vi "Load Interpolation Table.vi"(10 "File In":path, 11 "Object Name":string) -> (0 "error out":errorcluster, 1 "Reference":dbl[](array[numeric])=[40.0, -60.0, 0.0, 65.0, 0.0, 70.0, 0.0], 2 "Table":dbl[][](array[numeric]), 3 "File":path)   [LabVIEW 2013]
uses:
  ROS/Code/SubVIs/BaxterSide.ctl
  <vilib>/Utility/config.llb/Read Key (String).vi
  <vilib>/Utility/config.llb/NI_LVConfig.lvlib
panel:
  in  "side":T1=enum."right"
  # "Object X       ObjectY         ObjectZ        ObjectA         BaseX           BaseY           BaseZ          BaseA"
  # "Far Left"
  # "Far Right"
  # "Near Left"
  # "Near Right"
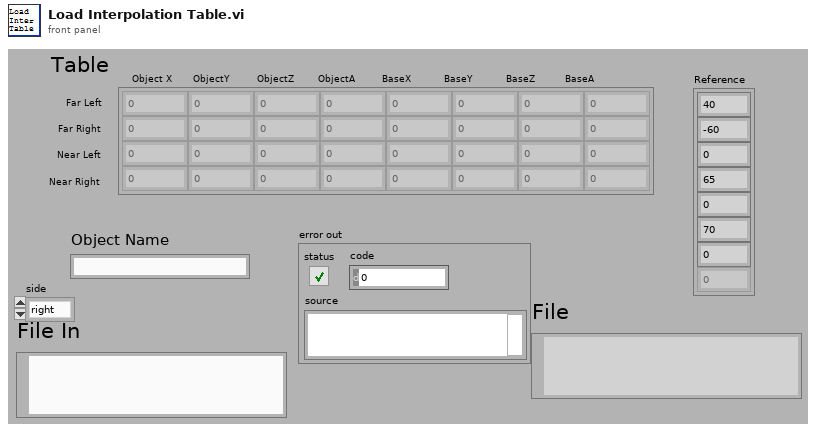
[diagram p1: front panel]
types:
  T1 = typedef "BaxterSide.ctl" = enum16{"left", "right"}
  T2 = typedef "NI_LVConfig.lvlib/Config Data RefNum.ctl" = refnum<k1>
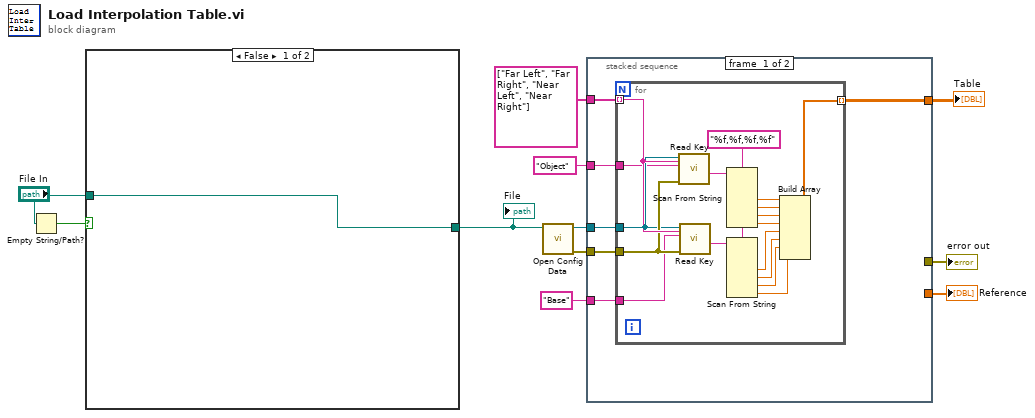
[diagram p0: block diagram]
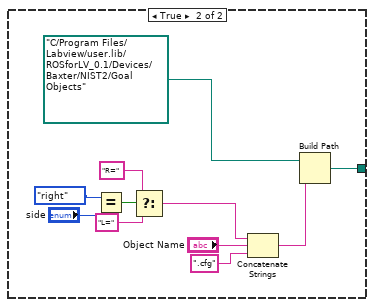
[diagram p2: hidden frame]
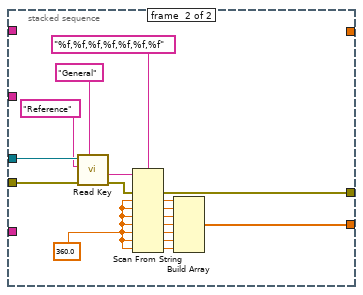
[diagram p3: hidden frame]
diagram:
  n1 = Empty String/Path?(string/path="File In") -> (empty?=w3:bool)
  n2 = case shown="False" w3 {
    tunnel: [w12 w23] -> w1
    tunnel: "File In" -> [w12 _]
    frame False {
    }
    frame True {
      n3 = Equal?(x=BaxterSide."right" ("Side"), y="side") -> (x = y?=w16:bool)
      n4 = Select(t="R=", s=w16, f="L=") -> (s? t:f=w15:string)
      n5 = Concatenate Strings(w15, "Object Name", ".cfg" ("replace string (\"\")")) -> (w20:string)
      n6 = Build Path(base path=path "C:/Program Files/Labview/user.lib/ROSforLV_0.1/Devices/Baxter/NIST2/Goal Objects", name or relative path=w20) -> (appended path=w23:path)
    }
  }
  "File" <- w1
  n7 = call <vilib>:"Open Config Data.vi"("configuration file path"=w1) -> ("error out"=w10:errorcluster, "refnum"=w11:T2)  [unwired: 8 in, 1 out]
  n8 = stacked-sequence {
    tunnel: w11 -> [w28 w63]
    tunnel: w10 -> [w29 w62]
    tunnel: [_ w50] -> w4
    tunnel: "Object" ("key") -> [w27 _]
    tunnel: "Base" ("key") -> [w26 _]
    tunnel: [_ w47] -> w6
    tunnel: string[] ["Far Left", "Far Right", "Near Left", "Near Right"] -> [w25 _]
    tunnel: [w24 _] -> w5
    frame #0 {
      n9 = for {
        tunnel: w25 -> [w43] mode=indexing
        tunnel: w29 -> [w42]
        tunnel: w28 -> [w41]
        tunnel: w27 -> [w40]
        tunnel: w26 -> [w39]
        tunnel: [w37] -> w24 mode=indexing
        w45 = "%f,%f,%f,%f" ("format string")
        n10 = call-poly <vilib>:"Read Key.vi"("section"=w43, "error in (no error)"=w42, "key"=w40, "refnum"=w41) -> ("value"=w46:string)  [unwired: 4 in, 3 out]
        n11 = call-poly <vilib>:"Read Key.vi"("section"=w43, "error in (no error)"=w42, "key"=w39, "refnum"=w41) -> ("value"=w44:string)  [unwired: 4 in, 3 out]
        n12 = Scan From String(format string=w45, input string=w46) -> (output 1=w38:dbl, output 2=w36:dbl, output 3=w35:dbl, output 4=w34:dbl)  [unwired: 6 in, 3 out]
        n13 = Scan From String(format string=w45, input string=w44) -> (output 1=w33:dbl, output 2=w32:dbl, output 3=w31:dbl, output 4=w30:dbl)  [unwired: 6 in, 3 out]
        n14 = Build Array(w38, w36, w35, w34, w33, w32, w31, w30) -> (w37:dbl[])
      }
    }
    frame #1 {
      w49 = 360.0 ("default value 1")
      n15 = call-poly <vilib>:"Read Key.vi"("section"="General", "error in (no error)"=w62, "key"="Reference", "refnum"=w63) -> ("error out"=w48:errorcluster, "value"=w60:string)  [unwired: 4 in, 2 out]
      n16 = Scan From String(format string="%f,%f,%f,%f,%f,%f,%f", input string=w60, error in=w48, default 1=w49, default 2=w49, default 3=w49, default 4=w49, default 5=w49, default 6=w49, default 7=w49) -> (error out=w47:errorcluster, output 1=w59:dbl, output 2=w58:dbl, output 3=w57:dbl, output 4=w56:dbl, output 5=w53:dbl, output 6=w52:dbl, output 7=w51:dbl)  [unwired: 1 in, 2 out]
      n17 = Build Array(w59, w58, w57, w56, w53, w52, w51) -> (w50:dbl[])
    }
  }
  "error out" <- w6
  "Reference" <- w4
  "Table" <- w5
